vi "Delimiter.vi"() -> (3 "Delimiter":string)   [LabVIEW 2023, in "SLL Environment Variable.lvlib"]
doc: "Assign the delimiter constant <B>(;)</B>"
uses:
  SLL Environment Variable.lvlib
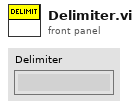
[diagram p1: front panel]
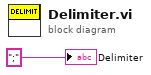
[diagram p0: block diagram]
diagram:
  "Delimiter" <- ";" ("String")
